vi "Sensors Parallel Read Test.vi"() -> ()   [LabVIEW 2009]
uses:
  <vilib>/userDefined/High Color/nirio_resource_hc.ctl
  <vilib>/rvi/interface/nirviCloseFPGA/nirviCloseFPGA.xnode
  <vilib>/rvi/interface/nirviOpenFPGA/nirviOpenFPGA.xnode
  FPGA Bitfiles/Q_IGVC_2010.lvproj_FPGA Target_FPGA_MAIN.vi.lvbitx
  <vilib>/Platform/TimedLoop/XDataNode/XDataNode.xnode
  <vilib>/Platform/TimedLoop/XDataNode/nitl_modes.ctl
  <vilib>/Platform/TimedLoop/XDataNode/XDNodeRunTimeDep.lvlib
  <vilib>/Platform/TimedLoop/XDataNode/wakeup.ctl
  <vilib>/Platform/TimedLoop/XDataNode/timing_clust.ctl
  <vilib>/Platform/TimedLoop/XDataNode/loadlvalarms.vi
  <vilib>/FPGAPlugInAG/cRIO-9113/nirviIntfOpen_cRIO-9113.vi
panel:
  out "Iteration Duration":i64
  out "Compass Bearing":dbl
  out "Waveform Graph":u16[](graph)
  out "Compass Loop Time":u32
  out "Buffer Not Empty":bool
  out "SICK Loop Time":u32
  out "Init Success":bool
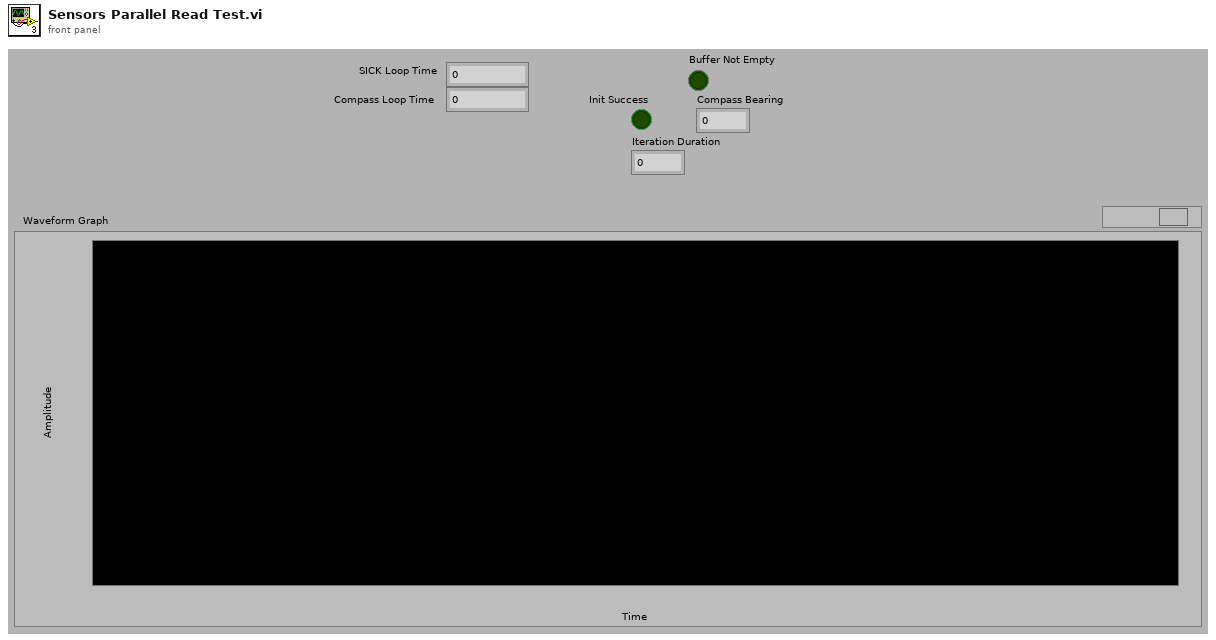
[diagram p1: front panel]
types:
  T1 = typedef "nirio_resource_hc.ctl" = tag
  T2 = typedef "XDNodeRunTimeDep.lvlib/timing_clust.ctl" = cluster{"Expected End [f-1]":u64, "Actual End [f-1]":u64, "Finished Late? [f-1]":bool, "Expected End [i-1]":u64, "Actual End [i-1]":u64, "Finished Late? [i-1]":bool, "Expected Start [i]":u64, "Actual Start [i]":u64, "Expected Start [f]":u64, "Actual Start [f]":u64, "Source Name":string, "Structure Name":string, "Period":i64, "Deadline":i64, "Offset":i64, "Start":i64, "Priority":i32, "Timeout":i32, "Mode":T3, "Wakeup Reason":T4, "Error":errorcluster, "Source Type":string, "Secondary Source Type":string, "Global End Time":u64, "Global Start Time":u64, "Frame Duration":u64, "Iteration Duration":u64, "Assigned CPU":i32, "I/O Scan Engine Mode":u32}
  T3 = typedef "XDNodeRunTimeDep.lvlib/nitl_modes.ctl" = enum32{"No Change", "Process missed periods, maintain original phase", "Discard missed periods, maintain original phase", "Process missed periods, ignore original phase", "Discard missed periods, ignore original phase"}
  T4 = typedef "XDNodeRunTimeDep.lvlib/wakeup.ctl" = enum32{"Normal", "Aborted", "Asynchronous wakeup", "Timing source error", "Timed loop error", "Timeout"}
  T5 = cluster{"signature":u8[], "vi signatures match":bool, "signature register address":u32, "reset register address":u32, "control register address":u32, "interrupt base address":u32, "Bitstream Version":u32, "DMA Configuration":cluster{"Name":string, "Depth":u32, "Write? (Deprecated:Use Implementation)":bool, "Physical Channel":u32, "Base Address":u32, "Data Width":u32, "Data Type":enum32{"Boolean", "I8", "I16", "I32", "I64", "U8", "U16", "U32", "U64", "FXP"}, "FXP Properties":variant, "Write Window Address":u32, "Implementation":enum16{"niFpgaTargetToHost", "niFpgaHostToTarget", "niFpgaPeerToPeerWriter", "niFpgaPeerToPeerReader", "niCoreTargetToHost", "niCoreHostToTarget"}, "Control Set":u32}[], "run when loaded?":bool, "reset register size in bits":u32, "compilation results xml":string}
  T6 = typedef "FPGA Main ref.ctl" = refnum<k20>
  T7 = typedef "SICK Array.ctl" = u16[]
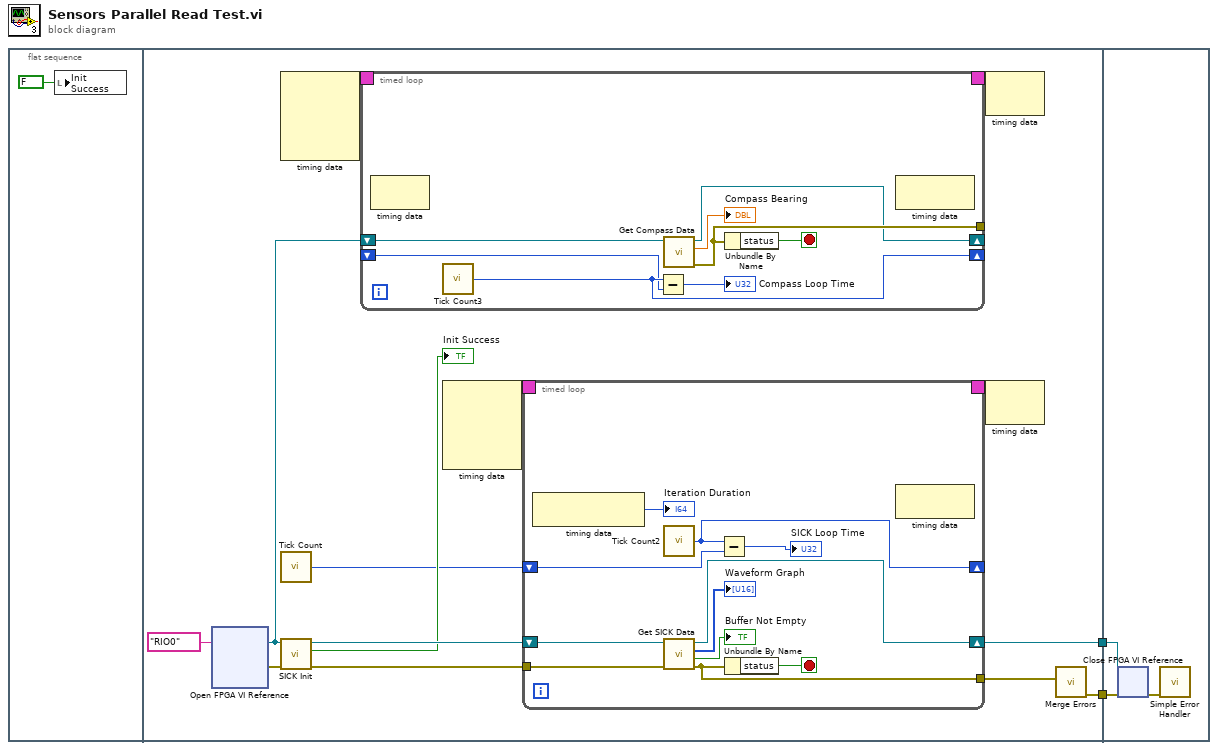
[diagram p0: block diagram]
diagram:
  n1 = flat-sequence {
    tunnel: [w17] -> w2
    tunnel: [w12] -> w1
    tunnel: w2 -> [w59]
    tunnel: w1 -> [w57]
    frame #0 {
      n2 = local write "Init Success"(FALSE ("all stop")) -> ()
    }
    frame #1 {
      n3 = xnode "Open FPGA VI Reference"("resource name"=T1 "RIO0") -> ("FPGA VI Reference Out"=w8:refnum<k20>, "error out"=w9:errorcluster)  [unwired: 1 in]
      n4 = node-c288() -> (w5:T2)  [unwired: 4 in]
      n5 = call "Tick Count"() -> ("Tick Count(uSec)"=w11:u32)
      n6 = call "SICK Init.vi"("error in"=w9, "FPGA_MAIN ref in"=w8) -> ("error out"=w14:errorcluster, "Init Success"=→"Init Success":bool, "FPGA_MAIN ref out"=w15:T6)  [unwired: 7 in]
      n7 = timed-loop {
        tunnel: [w25] -> _
        shift-right: [w23] -> _
        shift-left: w8 -> [w24]
        shift-right: [w22] -> _
        shift-left: _ -> [w20]
        timing: w5 -> [_]
        timing-out: [_] -> w4
        stop <- w19 stop-if-true
        n8 = node-c288() -> ()  [unwired: 1 in, 1 out]
        n9 = call "Tick Count3"() -> ("Tick Count(uSec)"=w22:u32)
        n10 = Subtract(x=w22, y=w20) -> (x-y=→"Compass Loop Time":u32)
        n11 = call "Get Compass Data.vi"("FPGA_MAIN ref in"=w24) -> ("error out"=w25:errorcluster, "Compass Bearing"=→"Compass Bearing":dbl, "FPGA_MAIN ref out"=w23:T6)  [unwired: 8 in]
        n12 = Unbundle By Name(w25) -> ("status"=w19:bool)
        n13 = node-c288() -> ()  [unwired: 1 in, 1 out]
      }
      n14 = node-c288() -> (w7:T2)  [unwired: 4 in]
      n15 = timed-loop {
        tunnel: [w40] -> w16
        tunnel: w14 -> [w38]
        shift-right: [w37] -> w12
        shift-left: w15 -> [w39]
        shift-right: [w36] -> _
        shift-left: w11 -> [w34]
        timing: w7 -> [_]
        timing-out: [_] -> w6
        stop <- w32 stop-if-true
        n16 = node-c288() -> (→"Iteration Duration":i64)  [unwired: 1 in]
        n17 = call "Tick Count2"() -> ("Tick Count(uSec)"=w36:u32)
        n18 = call "Get SICK Data.vi"("error in"=w38, "FPGA_MAIN ref in"=w39) -> ("error out"=w40:errorcluster, "Buffer Not Empty"=→"Buffer Not Empty":bool, "SICK Data"=→"Waveform Graph":T7, "FPGA_MAIN ref out"=w37:T6)  [unwired: 6 in]
        n19 = Subtract(x=w36, y=w34) -> (x-y=→"SICK Loop Time":u32)
        n20 = Unbundle By Name(w40) -> ("status"=w32:bool)
        n21 = node-c288() -> ()  [unwired: 1 in, 1 out]
      }
      n22 = node-c288(w4) -> ()  [unwired: 1 out]
      n23 = node-c288(w6) -> ()  [unwired: 1 out]
      n24 = call <vilib>:"Merge Errors.vi"("error in 2 (no error)"=w16) -> ("error out"=w17:errorcluster)  [unwired: 6 in]
    }
    frame #2 {
      n25 = xnode "Close FPGA VI Reference"("FPGA VI Reference In"=w57, "error in"=w59) -> ("error out"=w58:errorcluster)
      n26 = call <vilib>:"Simple Error Handler.vi"("error in (no error)"=w58) -> ()  [unwired: 4 in, 5 out]
    }
  }
